vi "source.vi"(4 "error in (no error)":errorcluster, 6 "modulation parameters in":T1={"modulation type"="QPSK", "pulse shaping parameters"={"modulation type"=enum."PSK", "pulse shaping filter"=enum."Root Raised Cos", "filter parameter"=0.5, "filter length (symbols)"=8}, "TX oversample\nfactor"=20, "packet length\n(bits)"=500, "number of data \nsymbols (derived)"=100, "TX sample rate"=0.0, "control information\nfor packet header/tail"={"Training Sequence"=[0.7071067811865475+0.7071067811865475i, 0.7071067811865475+0.7071067811865475i, 0.7071067811865475+0.7071067811865475i, -0.7071067811865475-0.7071067811865475i, -0.7071067811865475-0.7071067811865475i, -0.7071067811865475-0.7071067811865475i, 0.7071067811865475+0.7071067811865475i, -0.7071067811865475-0.7071067811865475i, -0.7071067811865475-0.7071067811865475i, 0.7071067811865475+0.7071067811865475i, -0.7071067811865475-0.7071067811865475i, 0.7071067811865475+0.7071067811865475i, 0.7071067811865475+0.7071067811865475i, 0.7071067811865475+0.7071067811865475i, -0.7071067811865475-0.7071067811865475i, -0.7071067811865475-0.7071067811865475i, -0.7071067811865475-0.7071067811865475i, 0.7071067811865475+0.7071067811865475i, -0.7071067811865475-0.7071067811865475i, -0.7071067811865475-0.7071067811865475i, 0.7071067811865475+0.7071067811865475i, -0.7071067811865475-0.7071067811865475i, 0.7071067811865475+0.7071067811865475i, 0.7071067811865475+0.7071067811865475i, 0.7071067811865475+0.7071067811865475i, -0.7071067811865475-0.7071067811865475i, -0.7071067811865475-0.7071067811865475i, -0.7071067811865475-0.7071067811865475i, 0.7071067811865475+0.7071067811865475i, -0.7071067811865475-0.7071067811865475i, -0.7071067811865475-0.7071067811865475i, 0.7071067811865475+0.7071067811865475i, -0.7071067811865475-0.7071067811865475i, 0.7071067811865475+0.7071067811865475i, 0.7071067811865475+0.7071067811865475i, 0.7071067811865475+0.7071067811865475i, -0.7071067811865475-0.7071067811865475i, -0.7071067811865475-0.7071067811865475i, -0.7071067811865475-0.7071067811865475i, 0.7071067811865475+0.7071067811865475i, -0.7071067811865475-0.7071067811865475i, -0.7071067811865475-0.7071067811865475i, 0.7071067811865475+0.7071067811865475i, -0.7071067811865475-0.7071067811865475i], "Zero Pad Length"=-2147483648, "Zero Pad Sequence"=[], "Training Sequence Type"="Barker Sequence-11"}} {"control information\nfor packet header/tail"."Training Sequence" format="%#_3p"; "TX sample rate" items=["100M"=100000000.0, "50M"=50000000.0, "33.3333M"=33333333.333333332, "25M"=25000000.0, "20M"=20000000.0, "16.6667M"=16666666.666666666, "14.2857M"=14285714.285714285, "12.5M"=12500000.0, "11.1111M"=11111111.111111112, "10M"=10000000.0, "9.09091M"=9090909.090909092, "8.33333M"=8333333.333333333, "7.69231M"=7692307.692307692, "7.14286M"=7142857.142857143, "6.66667M"=6666666.666666667, "6.25M"=6250000.0, "5.88235M"=5882352.94117647, "5.55556M"=5555555.555555556, "5.26316M"=5263157.894736842, "5M"=5000000.0, "4.7619M"=4761904.761904762, "4.54545M"=4545454.545454546, "4.34783M"=4347826.0869565215, "4.16667M"=4166666.6666666665, "4M"=4000000.0, "3.84615M"=3846153.846153846, "3.7037M"=3703703.703703704, "3.57143M"=3571428.5714285714, "3.44828M"=3448275.8620689656, "3.33333M"=3333333.3333333335, "3.22581M"=3225806.4516129033, "3.125M"=3125000.0, "3.0303M"=3030303.0303030303, "2.94118M"=2941176.470588235, "2.85714M"=2857142.8571428573, "2.77778M"=2777777.777777778, "2.7027M"=2702702.7027027025, "2.63158M"=2631578.947368421, "2.5641M"=2564102.564102564, "2.5M"=2500000.0, "2.43902M"=2439024.3902439023, "2.38095M"=2380952.380952381, "2.32558M"=2325581.395348837, "2.27273M"=2272727.272727273, "2.22222M"=2222222.222222222, "2.17391M"=2173913.0434782607, "2.12766M"=2127659.574468085, "2.08333M"=2083333.3333333333, "2.04082M"=2040816.3265306123, "2M"=2000000.0, "1.96078M"=1960784.3137254901, "1.92308M"=1923076.923076923, "1.88679M"=1886792.4528301887, "1.85185M"=1851851.851851852, "1.81818M"=1818181.8181818181, "1.78571M"=1785714.2857142857, "1.75439M"=1754385.9649122807, "1.72414M"=1724137.9310344828, "1.69492M"=1694915.2542372881, "1.66667M"=1666666.6666666667, "1.63934M"=1639344.262295082, "1.6129M"=1612903.2258064516, "1.5873M"=1587301.5873015872, "1.5625M"=1562500.0, "1.53846M"=1538461.5384615385, "1.51515M"=1515151.5151515151, "1.49254M"=1492537.3134328357, "1.47059M"=1470588.2352941176, "1.44928M"=1449275.3623188406, "1.42857M"=1428571.4285714286, "1.40845M"=1408450.704225352, "1.38889M"=1388888.888888889, "1.36986M"=1369863.01369863, "1.35135M"=1351351.3513513512, "1.33333M"=1333333.3333333333, "1.31579M"=1315789.4736842106, "1.2987M"=1298701.2987012987, "1.28205M"=1282051.282051282, "1.26582M"=1265822.7848101265, "1.25M"=1250000.0, "1.23457M"=1234567.9012345679, "1.21951M"=1219512.1951219512, "1.20482M"=1204819.2771084337, "1.19048M"=1190476.1904761905, "1.17647M"=1176470.5882352942, "1.16279M"=1162790.6976744186, "1.14943M"=1149425.287356322, "1.13636M"=1136363.6363636365, "1.1236M"=1123595.5056179776, "1.11111M"=1111111.111111111, "1.0989M"=1098901.0989010988, "1.08696M"=1086956.5217391304, "1.07527M"=1075268.817204301, "1.06383M"=1063829.7872340425, "1.05263M"=1052631.5789473683, "1.04167M"=1041666.6666666666, "1.03093M"=1030927.8350515463, "1.02041M"=1020408.1632653062, "1.0101M"=1010101.0101010101, "1M"=1000000.0, "990.099k"=990099.0099009901, "980.392k"=980392.1568627451, "970.874k"=970873.786407767, "961.538k"=961538.4615384615, "952.381k"=952380.9523809524, "943.396k"=943396.2264150943, "934.579k"=934579.4392523364, "925.926k"=925925.925925926, "917.431k"=917431.1926605505, "909.091k"=909090.9090909091, "900.901k"=900900.900900901, "892.857k"=892857.1428571428, "884.956k"=884955.7522123894, "877.193k"=877192.9824561403, "869.565k"=869565.2173913043, "862.069k"=862068.9655172414, "854.701k"=854700.8547008547, "847.458k"=847457.6271186441, "840.336k"=840336.1344537815, "833.333k"=833333.3333333334, "826.446k"=826446.2809917355, "819.672k"=819672.131147541, "813.008k"=813008.1300813009, "806.452k"=806451.6129032258, "800k"=800000.0, "793.651k"=793650.7936507936, "787.402k"=787401.5748031496, "781.25k"=781250.0, "769.231k"=769230.7692307692, "757.576k"=757575.7575757576, "746.269k"=746268.6567164179, "735.294k"=735294.1176470588, "724.638k"=724637.6811594203, "714.286k"=714285.7142857143, "704.225k"=704225.352112676, "694.444k"=694444.4444444445, "684.932k"=684931.506849315, "675.676k"=675675.6756756756, "666.667k"=666666.6666666666, "657.895k"=657894.7368421053, "649.351k"=649350.6493506493, "641.026k"=641025.641025641, "632.911k"=632911.3924050633, "625k"=625000.0, "617.284k"=617283.9506172839, "609.756k"=609756.0975609756, "602.41k"=602409.6385542168, "595.238k"=595238.0952380953, "588.235k"=588235.2941176471, "581.395k"=581395.3488372093, "574.713k"=574712.643678161, "568.182k"=568181.8181818182, "561.798k"=561797.7528089888, "555.556k"=555555.5555555555, "549.451k"=549450.5494505494, "543.478k"=543478.2608695652, "537.634k"=537634.4086021505, "531.915k"=531914.8936170213, "526.316k"=526315.7894736842, "520.833k"=520833.3333333333, "515.464k"=515463.91752577317, "510.204k"=510204.0816326531, "505.051k"=505050.50505050505, "500k"=500000.0, "495.05k"=495049.50495049503, "490.196k"=490196.07843137253, "485.437k"=485436.8932038835, "480.769k"=480769.23076923075, "476.19k"=476190.4761904762, "471.698k"=471698.11320754717, "467.29k"=467289.7196261682, "462.963k"=462962.962962963, "458.716k"=458715.59633027524, "454.545k"=454545.45454545453, "450.45k"=450450.4504504505, "446.429k"=446428.5714285714, "442.478k"=442477.8761061947, "438.596k"=438596.49122807017, "434.783k"=434782.60869565216, "431.034k"=431034.4827586207, "427.35k"=427350.4273504274, "423.729k"=423728.81355932204, "420.168k"=420168.06722689077, "416.667k"=416666.6666666667, "413.223k"=413223.14049586776, "409.836k"=409836.0655737705, "406.504k"=406504.0650406504, "403.226k"=403225.8064516129, "400k"=400000.0, "396.825k"=396825.3968253968, "393.701k"=393700.7874015748, "390.625k"=390625.0, "384.615k"=384615.3846153846, "378.788k"=378787.8787878788, "373.134k"=373134.32835820894, "367.647k"=367647.0588235294, "362.319k"=362318.84057971014, "357.143k"=357142.85714285716, "352.113k"=352112.676056338, "347.222k"=347222.22222222225, "342.466k"=342465.7534246575, "337.838k"=337837.8378378378, "333.333k"=333333.3333333333, "328.947k"=328947.36842105264, "324.675k"=324675.32467532466, "320.513k"=320512.8205128205, "316.456k"=316455.69620253163, "312.5k"=312500.0, "308.642k"=308641.97530864197, "304.878k"=304878.0487804878, "301.205k"=301204.8192771084, "297.619k"=297619.04761904763, "294.118k"=294117.64705882355, "290.698k"=290697.67441860464, "287.356k"=287356.3218390805, "284.091k"=284090.9090909091, "280.899k"=280898.8764044944, "277.778k"=277777.77777777775, "274.725k"=274725.2747252747, "271.739k"=271739.1304347826, "268.817k"=268817.20430107525, "265.957k"=265957.44680851063, "263.158k"=263157.8947368421, "260.417k"=260416.66666666666, "257.732k"=257731.95876288658, "255.102k"=255102.04081632654, "252.525k"=252525.25252525252, "250k"=250000.0, "247.525k"=247524.75247524751, "245.098k"=245098.03921568627, "242.718k"=242718.44660194175, "240.385k"=240384.61538461538, "238.095k"=238095.2380952381, "235.849k"=235849.05660377358, "233.645k"=233644.8598130841, "231.481k"=231481.4814814815, "229.358k"=229357.79816513762, "227.273k"=227272.72727272726, "225.225k"=225225.22522522524, "223.214k"=223214.2857142857, "221.239k"=221238.93805309734, "219.298k"=219298.24561403508, "217.391k"=217391.30434782608, "215.517k"=215517.24137931035, "213.675k"=213675.2136752137, "211.864k"=211864.40677966102, "210.084k"=210084.03361344538, "208.333k"=208333.33333333334, "206.612k"=206611.57024793388, "204.918k"=204918.03278688525, "203.252k"=203252.0325203252, "201.613k"=201612.90322580645, "200k"=200000.0, "198.413k"=198412.6984126984, "196.85k"=196850.3937007874, "195.312k"=195312.5]}) -> (0 "error out":errorcluster, 2 "modulation parameters out":T1={"modulation type"="QPSK", "pulse shaping parameters"={"modulation type"=enum."PSK", "pulse shaping filter"=enum."Root Raised Cos", "filter parameter"=0.5, "filter length (symbols)"=8}, "TX oversample\nfactor"=20, "packet length\n(bits)"=500, "number of data \nsymbols (derived)"=100, "TX sample rate"=0.0, "control information\nfor packet header/tail"={"Training Sequence"=[0.7071067811865475+0.7071067811865475i, 0.7071067811865475+0.7071067811865475i, 0.7071067811865475+0.7071067811865475i, -0.7071067811865475-0.7071067811865475i, -0.7071067811865475-0.7071067811865475i, -0.7071067811865475-0.7071067811865475i, 0.7071067811865475+0.7071067811865475i, -0.7071067811865475-0.7071067811865475i, -0.7071067811865475-0.7071067811865475i, 0.7071067811865475+0.7071067811865475i, -0.7071067811865475-0.7071067811865475i, 0.7071067811865475+0.7071067811865475i, 0.7071067811865475+0.7071067811865475i, 0.7071067811865475+0.7071067811865475i, -0.7071067811865475-0.7071067811865475i, -0.7071067811865475-0.7071067811865475i, -0.7071067811865475-0.7071067811865475i, 0.7071067811865475+0.7071067811865475i, -0.7071067811865475-0.7071067811865475i, -0.7071067811865475-0.7071067811865475i, 0.7071067811865475+0.7071067811865475i, -0.7071067811865475-0.7071067811865475i, 0.7071067811865475+0.7071067811865475i, 0.7071067811865475+0.7071067811865475i, 0.7071067811865475+0.7071067811865475i, -0.7071067811865475-0.7071067811865475i, -0.7071067811865475-0.7071067811865475i, -0.7071067811865475-0.7071067811865475i, 0.7071067811865475+0.7071067811865475i, -0.7071067811865475-0.7071067811865475i, -0.7071067811865475-0.7071067811865475i, 0.7071067811865475+0.7071067811865475i, -0.7071067811865475-0.7071067811865475i, 0.7071067811865475+0.7071067811865475i, 0.7071067811865475+0.7071067811865475i, 0.7071067811865475+0.7071067811865475i, -0.7071067811865475-0.7071067811865475i, -0.7071067811865475-0.7071067811865475i, -0.7071067811865475-0.7071067811865475i, 0.7071067811865475+0.7071067811865475i, -0.7071067811865475-0.7071067811865475i, -0.7071067811865475-0.7071067811865475i, 0.7071067811865475+0.7071067811865475i, -0.7071067811865475-0.7071067811865475i], "Zero Pad Length"=-2147483648, "Zero Pad Sequence"=[], "Training Sequence Type"="Barker Sequence-11"}} {"control information\nfor packet header/tail"."Training Sequence" format="%#_3p"; "TX sample rate" items=["100M"=100000000.0, "50M"=50000000.0, "33.3333M"=33333333.333333332, "25M"=25000000.0, "20M"=20000000.0, "16.6667M"=16666666.666666666, "14.2857M"=14285714.285714285, "12.5M"=12500000.0, "11.1111M"=11111111.111111112, "10M"=10000000.0, "9.09091M"=9090909.090909092, "8.33333M"=8333333.333333333, "7.69231M"=7692307.692307692, "7.14286M"=7142857.142857143, "6.66667M"=6666666.666666667, "6.25M"=6250000.0, "5.88235M"=5882352.94117647, "5.55556M"=5555555.555555556, "5.26316M"=5263157.894736842, "5M"=5000000.0, "4.7619M"=4761904.761904762, "4.54545M"=4545454.545454546, "4.34783M"=4347826.0869565215, "4.16667M"=4166666.6666666665, "4M"=4000000.0, "3.84615M"=3846153.846153846, "3.7037M"=3703703.703703704, "3.57143M"=3571428.5714285714, "3.44828M"=3448275.8620689656, "3.33333M"=3333333.3333333335, "3.22581M"=3225806.4516129033, "3.125M"=3125000.0, "3.0303M"=3030303.0303030303, "2.94118M"=2941176.470588235, "2.85714M"=2857142.8571428573, "2.77778M"=2777777.777777778, "2.7027M"=2702702.7027027025, "2.63158M"=2631578.947368421, "2.5641M"=2564102.564102564, "2.5M"=2500000.0, "2.43902M"=2439024.3902439023, "2.38095M"=2380952.380952381, "2.32558M"=2325581.395348837, "2.27273M"=2272727.272727273, "2.22222M"=2222222.222222222, "2.17391M"=2173913.0434782607, "2.12766M"=2127659.574468085, "2.08333M"=2083333.3333333333, "2.04082M"=2040816.3265306123, "2M"=2000000.0, "1.96078M"=1960784.3137254901, "1.92308M"=1923076.923076923, "1.88679M"=1886792.4528301887, "1.85185M"=1851851.851851852, "1.81818M"=1818181.8181818181, "1.78571M"=1785714.2857142857, "1.75439M"=1754385.9649122807, "1.72414M"=1724137.9310344828, "1.69492M"=1694915.2542372881, "1.66667M"=1666666.6666666667, "1.63934M"=1639344.262295082, "1.6129M"=1612903.2258064516, "1.5873M"=1587301.5873015872, "1.5625M"=1562500.0, "1.53846M"=1538461.5384615385, "1.51515M"=1515151.5151515151, "1.49254M"=1492537.3134328357, "1.47059M"=1470588.2352941176, "1.44928M"=1449275.3623188406, "1.42857M"=1428571.4285714286, "1.40845M"=1408450.704225352, "1.38889M"=1388888.888888889, "1.36986M"=1369863.01369863, "1.35135M"=1351351.3513513512, "1.33333M"=1333333.3333333333, "1.31579M"=1315789.4736842106, "1.2987M"=1298701.2987012987, "1.28205M"=1282051.282051282, "1.26582M"=1265822.7848101265, "1.25M"=1250000.0, "1.23457M"=1234567.9012345679, "1.21951M"=1219512.1951219512, "1.20482M"=1204819.2771084337, "1.19048M"=1190476.1904761905, "1.17647M"=1176470.5882352942, "1.16279M"=1162790.6976744186, "1.14943M"=1149425.287356322, "1.13636M"=1136363.6363636365, "1.1236M"=1123595.5056179776, "1.11111M"=1111111.111111111, "1.0989M"=1098901.0989010988, "1.08696M"=1086956.5217391304, "1.07527M"=1075268.817204301, "1.06383M"=1063829.7872340425, "1.05263M"=1052631.5789473683, "1.04167M"=1041666.6666666666, "1.03093M"=1030927.8350515463, "1.02041M"=1020408.1632653062, "1.0101M"=1010101.0101010101, "1M"=1000000.0, "990.099k"=990099.0099009901, "980.392k"=980392.1568627451, "970.874k"=970873.786407767, "961.538k"=961538.4615384615, "952.381k"=952380.9523809524, "943.396k"=943396.2264150943, "934.579k"=934579.4392523364, "925.926k"=925925.925925926, "917.431k"=917431.1926605505, "909.091k"=909090.9090909091, "900.901k"=900900.900900901, "892.857k"=892857.1428571428, "884.956k"=884955.7522123894, "877.193k"=877192.9824561403, "869.565k"=869565.2173913043, "862.069k"=862068.9655172414, "854.701k"=854700.8547008547, "847.458k"=847457.6271186441, "840.336k"=840336.1344537815, "833.333k"=833333.3333333334, "826.446k"=826446.2809917355, "819.672k"=819672.131147541, "813.008k"=813008.1300813009, "806.452k"=806451.6129032258, "800k"=800000.0, "793.651k"=793650.7936507936, "787.402k"=787401.5748031496, "781.25k"=781250.0, "769.231k"=769230.7692307692, "757.576k"=757575.7575757576, "746.269k"=746268.6567164179, "735.294k"=735294.1176470588, "724.638k"=724637.6811594203, "714.286k"=714285.7142857143, "704.225k"=704225.352112676, "694.444k"=694444.4444444445, "684.932k"=684931.506849315, "675.676k"=675675.6756756756, "666.667k"=666666.6666666666, "657.895k"=657894.7368421053, "649.351k"=649350.6493506493, "641.026k"=641025.641025641, "632.911k"=632911.3924050633, "625k"=625000.0, "617.284k"=617283.9506172839, "609.756k"=609756.0975609756, "602.41k"=602409.6385542168, "595.238k"=595238.0952380953, "588.235k"=588235.2941176471, "581.395k"=581395.3488372093, "574.713k"=574712.643678161, "568.182k"=568181.8181818182, "561.798k"=561797.7528089888, "555.556k"=555555.5555555555, "549.451k"=549450.5494505494, "543.478k"=543478.2608695652, "537.634k"=537634.4086021505, "531.915k"=531914.8936170213, "526.316k"=526315.7894736842, "520.833k"=520833.3333333333, "515.464k"=515463.91752577317, "510.204k"=510204.0816326531, "505.051k"=505050.50505050505, "500k"=500000.0, "495.05k"=495049.50495049503, "490.196k"=490196.07843137253, "485.437k"=485436.8932038835, "480.769k"=480769.23076923075, "476.19k"=476190.4761904762, "471.698k"=471698.11320754717, "467.29k"=467289.7196261682, "462.963k"=462962.962962963, "458.716k"=458715.59633027524, "454.545k"=454545.45454545453, "450.45k"=450450.4504504505, "446.429k"=446428.5714285714, "442.478k"=442477.8761061947, "438.596k"=438596.49122807017, "434.783k"=434782.60869565216, "431.034k"=431034.4827586207, "427.35k"=427350.4273504274, "423.729k"=423728.81355932204, "420.168k"=420168.06722689077, "416.667k"=416666.6666666667, "413.223k"=413223.14049586776, "409.836k"=409836.0655737705, "406.504k"=406504.0650406504, "403.226k"=403225.8064516129, "400k"=400000.0, "396.825k"=396825.3968253968, "393.701k"=393700.7874015748, "390.625k"=390625.0, "384.615k"=384615.3846153846, "378.788k"=378787.8787878788, "373.134k"=373134.32835820894, "367.647k"=367647.0588235294, "362.319k"=362318.84057971014, "357.143k"=357142.85714285716, "352.113k"=352112.676056338, "347.222k"=347222.22222222225, "342.466k"=342465.7534246575, "337.838k"=337837.8378378378, "333.333k"=333333.3333333333, "328.947k"=328947.36842105264, "324.675k"=324675.32467532466, "320.513k"=320512.8205128205, "316.456k"=316455.69620253163, "312.5k"=312500.0, "308.642k"=308641.97530864197, "304.878k"=304878.0487804878, "301.205k"=301204.8192771084, "297.619k"=297619.04761904763, "294.118k"=294117.64705882355, "290.698k"=290697.67441860464, "287.356k"=287356.3218390805, "284.091k"=284090.9090909091, "280.899k"=280898.8764044944, "277.778k"=277777.77777777775, "274.725k"=274725.2747252747, "271.739k"=271739.1304347826, "268.817k"=268817.20430107525, "265.957k"=265957.44680851063, "263.158k"=263157.8947368421, "260.417k"=260416.66666666666, "257.732k"=257731.95876288658, "255.102k"=255102.04081632654, "252.525k"=252525.25252525252, "250k"=250000.0, "247.525k"=247524.75247524751, "245.098k"=245098.03921568627, "242.718k"=242718.44660194175, "240.385k"=240384.61538461538, "238.095k"=238095.2380952381, "235.849k"=235849.05660377358, "233.645k"=233644.8598130841, "231.481k"=231481.4814814815, "229.358k"=229357.79816513762, "227.273k"=227272.72727272726, "225.225k"=225225.22522522524, "223.214k"=223214.2857142857, "221.239k"=221238.93805309734, "219.298k"=219298.24561403508, "217.391k"=217391.30434782608, "215.517k"=215517.24137931035, "213.675k"=213675.2136752137, "211.864k"=211864.40677966102, "210.084k"=210084.03361344538, "208.333k"=208333.33333333334, "206.612k"=206611.57024793388, "204.918k"=204918.03278688525, "203.252k"=203252.0325203252, "201.613k"=201612.90322580645, "200k"=200000.0, "198.413k"=198412.6984126984, "196.85k"=196850.3937007874, "195.312k"=195312.5]}, 3 "output bit stream":u8[](array[numeric]))   [LabVIEW 2013]
uses:
  QAM_Decode/TypeDefine/tx_modulation params.ctl
  <vilib>/addons/Modulation/Digital/General/MT Generate Bits (Galois, PN Order).vi
  <vilib>/addons/Modulation/niDMT.lvlib
panel:
  # "Generate random bit sequence of size length"
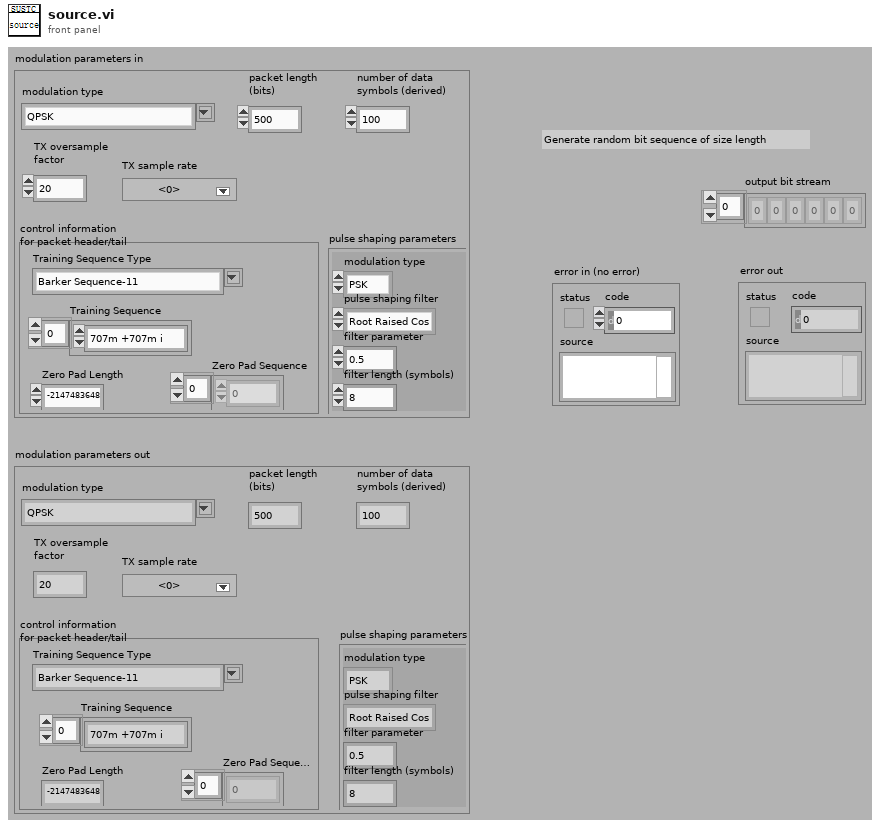
[diagram p1: front panel]
types:
  T1 = typedef "tx_modulation params.ctl" = cluster{"modulation type":string, "pulse shaping parameters":cluster{"modulation type":enum16{"FSK", "PSK", "QAM", "MSK", "PAM", "ASK"}, "pulse shaping filter":enum16{"none", "Raised Cosine", "Root Raised Cos", "Gaussian"}, "filter parameter":dbl, "filter length (symbols)":i32}, "TX oversample\nfactor":i32, "packet length\n(bits)":i32, "number of data \nsymbols (derived)":i32, "TX sample rate":dbl, "control information\nfor packet header/tail":cluster{"Training Sequence":cdb[], "Zero Pad Length":i32, "Zero Pad Sequence":cdb[], "Training Sequence Type":string}}
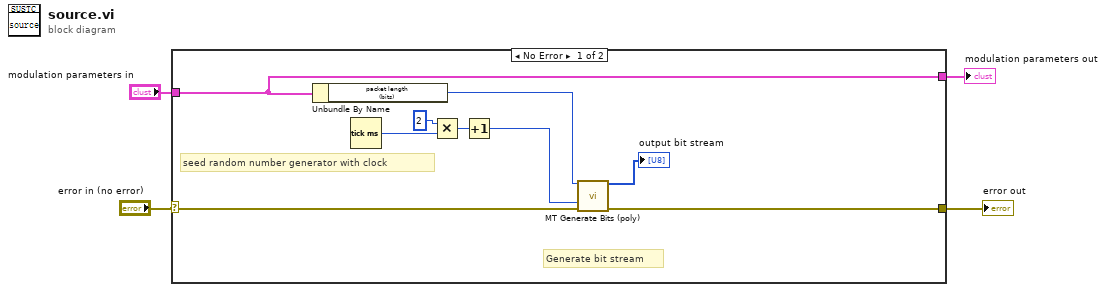
[diagram p0: block diagram]
diagram:
  n1 = case shown="No Error" "error in (no error)" {
    selector: "error in (no error)" -> [w6 w15]
    tunnel: [w8 w15] -> w4
    tunnel: [w5 w14] -> w2
    tunnel: "modulation parameters in" -> [w5 w14]
    frame No Error {
      # "Generate bit stream"
      # "seed random number generator with clock"
      n2 = Unbundle By Name(w5) -> ("packet length\n(bits)"=w7:i32)
      n3 = Tick Count (ms)() -> (millisecond timer value=w10:u32)
      n4 = Multiply(x=u32 2, y=w10) -> (x*y=w12:u32)
      n5 = Increment(x=w12) -> (x+1=w13:u32)
      n6 = call-poly <vilib>:"MT Generate Bits (poly).vi"("total bits (128)"=w7, "seed in (0xD6BF7DF2)"=w13, "error in (no error)"=w6) -> ("output bit stream"=→"output bit stream":i8[], "error out"=w8:errorcluster)  [unwired: 10 in, 1 out]
    }
    frame Error {
    }
  }
  "error out" <- w4
  "modulation parameters out" <- w2
